vi "drop_chunks.vi"(5 "hyper_table_name":string, 7 "connection_reference":T3, 8 "error in (no error)":errorcluster, 9 "chunk_options":T2 {"newer_than" format="%<%H:%M:%S>t"}, 10 "older_than":dbl format="%<%H:%M:%S>t", 11 "time_type":T1=enum."interval") -> (0 "error out":errorcluster, 3 "chunks_dropped []":string[](array[string]))   [LabVIEW 2015, in "lv-timescaledb.lvlib"]
uses:
  lv-timescaledb.lvlib
  <vilib>/addons/database/Connection.llb/Conn ObjectReference.ctl
  _controls/drop_chunk_options.ctl
  _controls/time_type.ctl
  <vilib>/addons/database/Command.llb/Cmd Execute.vi
  <vilib>/addons/database/Recordset.llb/Rec Fetch Recordset Data (CR).vi
  <vilib>/addons/database/Recordset.llb/Rec Destroy - Command.vi
  <vilib>/addons/database/Command.llb/Cmd Delete.vi
  <vilib>/addons/database/NI_Database_API.lvlib
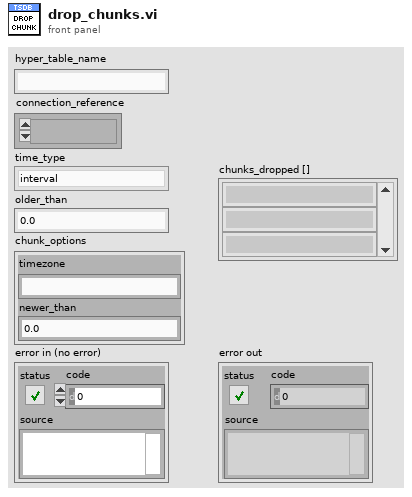
[diagram p1: front panel]
types:
  T1 = typedef "lv-timescaledb.lvlib/time_type.ctl" = enum16{"<time_type>", "interval", "timestamp", "timestamp_with_timezone", "<null>"}
  T2 = typedef "lv-timescaledb.lvlib/drop_chunk_options.ctl" = cluster{"timezone":string, "newer_than":dbl}
  T3 = typedef "NI_Database_API.lvlib/Conn ObjectReference.ctl" = refnum<k1>
  T4 = typedef "NI_Database_API.lvlib/DB Tools Parameter Info.ctl" = cluster{"parameter name":string, "type":T5, "direction":T6, "value":variant}
  T5 = typedef "NI_Database_API.lvlib/DB Tools DataTypes.ctl" = enum16{"String", "Long (I32)", "Single (SGL)", "Double (DBL)", "Date/Time", "Binary"}
  T6 = typedef "NI_Database_API.lvlib/DB Tools Parameter Dir.ctl" = enum32{"Input", "Output", "Input/Output", "Return Value"}
  T7 = cluster{"timezone":string, "postgres_date":string}
  T8 = typedef "NI_Database_API.lvlib/Cmd ObjectReference.ctl" = refnum<k1>
  T9 = typedef "NI_Database_API.lvlib/Cmd-Rec Object Reference.ctl" = refnum<k1>
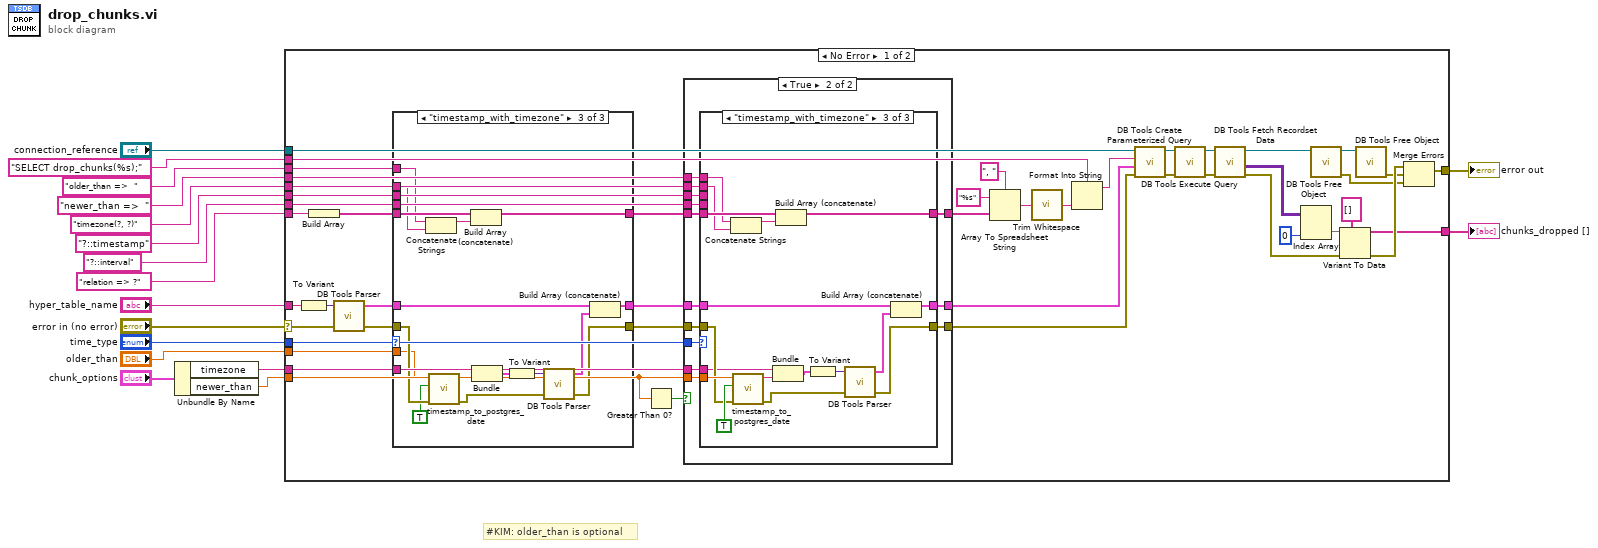
[diagram p0: block diagram]
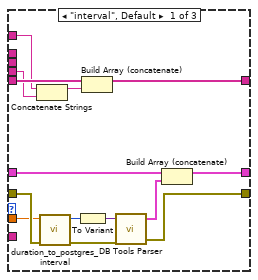
[diagram p2: hidden frame]
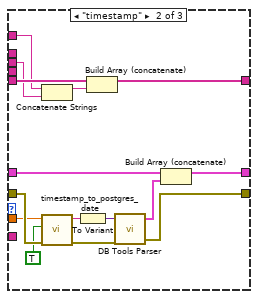
[diagram p3: hidden frame]
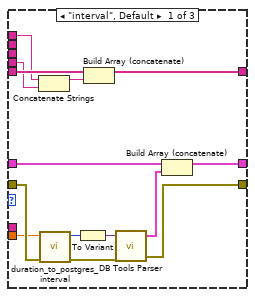
[diagram p5: hidden frame]
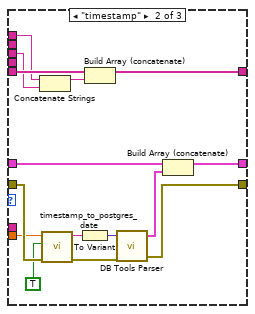
[diagram p6: hidden frame]
diagram:
  # "#KIM: older_than is optional"
  n1 = Unbundle By Name("chunk_options") -> ("timezone"=w1:string, "newer_than"=w9:dbl)
  n2 = case shown="No Error" "error in (no error)" {
    selector: "error in (no error)" -> [w45 w172]
    tunnel: "connection_reference" -> [w50 _]
    tunnel: [w61 w172] -> w15
    tunnel: [w47 _] -> w14
    tunnel: "hyper_table_name" -> [w44 _]
    tunnel: "time_type" -> [w25 _]
    tunnel: "older_than" -> [w40 _]
    tunnel: w9 -> [w32 _]
    tunnel: "SELECT drop_chunks(%s);" -> [w39 _]
    tunnel: "relation => ?" -> [w31 _]
    tunnel: "?::interval" -> [w20 _]
    tunnel: "?::timestamp" -> [w22 _]
    tunnel: "timezone(?, ?)" -> [w19 _]
    tunnel: "newer_than =>  " -> [w23 _]
    tunnel: "older_than =>  " -> [w24 _]
    tunnel: w1 -> [w18 _]
    frame No Error {
      n3 = To Variant(anything=w44) -> (Variant=w43:variant)
      n4 = Build Array(w31) -> (w30:string[])
      n5 = call <vilib>:"DB Tools Parser.vi"("error in (no error)"=w45, "variant"=w43) -> ("error out"=w41:errorcluster, "parameters"=w42:T4[])  [unwired: 2 in]
      n6 = case shown="\"timestamp_with_timezone\"" w25 {
        tunnel: w42 -> [w72 w84 w102]
        tunnel: w41 -> [w77 w92 w109]
        tunnel: w40 -> [w76 w91 w108]
        tunnel: [w71 w85 w103] -> w34
        tunnel: [w69 w83 w101] -> w63
        tunnel: w30 -> [w68 w81 w99]
        tunnel: [w67 w80 w98] -> w29
        tunnel: w24 -> [w64 w79 w97]
        tunnel: w20 -> [w65 _ _]
        tunnel: w22 -> [_ w78 _]
        tunnel: w18 -> [_ _ w93]
        tunnel: w19 -> [_ _ w96]
        frame "interval", Default {
          n7 = Concatenate Strings(w64, w65) -> (w66:string)
          n8 = call "duration_to_postgres_interval.vi"("error in (no error)"=w77, "interval"=w76) -> ("error out"=w74:errorcluster, "millisecond"=w75:i32)  [unwired: 8 in]
          n9 = To Variant(anything=w75) -> (Variant=w73:variant)
          n10 = Build Array (concatenate)(w68, w66) -> (w67:string[])
          n11 = call <vilib>:"DB Tools Parser.vi"("error in (no error)"=w74, "variant"=w73) -> ("error out"=w69:errorcluster, "parameters"=w70:T4[])  [unwired: 2 in]
          n12 = Build Array (concatenate)(w72, w70) -> (w71:T4[])
        }
        frame "timestamp" {
          n13 = Concatenate Strings(w79, w78) -> (w82:string)
          n14 = call "timestamp_to_postgres_date.vi"("error in (no error)"=w92, "utc"=TRUE, "date_time"=w91) -> ("error out"=w88:errorcluster, "postgres_date"=w89:string)  [unwired: 7 in]
          n15 = To Variant(anything=w89) -> (Variant=w87:variant)
          n16 = Build Array (concatenate)(w81, w82) -> (w80:string[])
          n17 = call <vilib>:"DB Tools Parser.vi"("error in (no error)"=w88, "variant"=w87) -> ("error out"=w83:errorcluster, "parameters"=w86:T4[])  [unwired: 2 in]
          n18 = Build Array (concatenate)(w84, w86) -> (w85:T4[])
        }
        frame "timestamp_with_timezone" {
          n19 = Concatenate Strings(w97, w96) -> (w100:string)
          n20 = call "timestamp_to_postgres_date.vi"("error in (no error)"=w109, "utc"=TRUE, "date_time"=w108) -> ("error out"=w106:errorcluster, "postgres_date"=w94:string)  [unwired: 7 in]
          n21 = Build Array (concatenate)(w99, w100) -> (w98:string[])
          n22 = Bundle("timezone"=w93, "postgres_date"=w94) -> (w95:T7)  [unwired: 1 in]
          n23 = To Variant(anything=w95) -> (Variant=w105:variant)
          n24 = call <vilib>:"DB Tools Parser.vi"("error in (no error)"=w106, "variant"=w105) -> ("error out"=w101:errorcluster, "parameters"=w104:T4[])  [unwired: 2 in]
          n25 = Build Array (concatenate)(w102, w104) -> (w103:T4[])
        }
      }
      n26 = Greater Than 0?(x=w32) -> (x > 0?=w27:bool)
      n27 = case shown="True" w27 {
        tunnel: w25 -> [_ w125]
        tunnel: w34 -> [w111 w124]
        tunnel: [w111 w123] -> w33
        tunnel: w63 -> [w110 w122]
        tunnel: w32 -> [_ w121]
        tunnel: w29 -> [w112 w120]
        tunnel: [w112 w116] -> w28
        tunnel: [w110 w119] -> w26
        tunnel: w23 -> [_ w118]
        tunnel: w22 -> [_ w117]
        tunnel: w20 -> [_ w115]
        tunnel: w19 -> [_ w114]
        tunnel: w18 -> [_ w113]
        frame False {
        }
        frame True {
          n28 = case shown="\"timestamp_with_timezone\"" w125 {
            tunnel: w121 -> [w138 w153 w171]
            tunnel: [w134 w147 w166] -> w123
            tunnel: [w127 w146 w165] -> w119
            tunnel: w124 -> [w128 w145 w163]
            tunnel: w122 -> [w139 w154 w164]
            tunnel: w120 -> [w131 w143 w161]
            tunnel: w118 -> [w129 w142 w160]
            tunnel: w117 -> [_ w140 _]
            tunnel: [w130 w141 w159] -> w116
            tunnel: w115 -> [w126 _ _]
            tunnel: w114 -> [_ _ w158]
            tunnel: w113 -> [_ _ w155]
            frame "interval", Default {
              n29 = Concatenate Strings(w129, w126) -> (w132:string)
              n30 = call "duration_to_postgres_interval.vi"("error in (no error)"=w139, "interval"=w138) -> ("error out"=w136:errorcluster, "millisecond"=w137:i32)  [unwired: 8 in]
              n31 = To Variant(anything=w137) -> (Variant=w135:variant)
              n32 = Build Array (concatenate)(w131, w132) -> (w130:string[])
              n33 = call <vilib>:"DB Tools Parser.vi"("error in (no error)"=w136, "variant"=w135) -> ("error out"=w127:errorcluster, "parameters"=w133:T4[])  [unwired: 2 in]
              n34 = Build Array (concatenate)(w128, w133) -> (w134:T4[])
            }
            frame "timestamp" {
              n35 = Concatenate Strings(w142, w140) -> (w144:string)
              n36 = call "timestamp_to_postgres_date.vi"("error in (no error)"=w154, "utc"=TRUE, "date_time"=w153) -> ("error out"=w150:errorcluster, "postgres_date"=w151:string)  [unwired: 7 in]
              n37 = To Variant(anything=w151) -> (Variant=w149:variant)
              n38 = Build Array (concatenate)(w143, w144) -> (w141:string[])
              n39 = call <vilib>:"DB Tools Parser.vi"("error in (no error)"=w150, "variant"=w149) -> ("error out"=w146:errorcluster, "parameters"=w148:T4[])  [unwired: 2 in]
              n40 = Build Array (concatenate)(w145, w148) -> (w147:T4[])
            }
            frame "timestamp_with_timezone" {
              n41 = Concatenate Strings(w160, w158) -> (w162:string)
              n42 = call "timestamp_to_postgres_date.vi"("error in (no error)"=w164, "utc"=TRUE, "date_time"=w171) -> ("error out"=w169:errorcluster, "postgres_date"=w157:string)  [unwired: 7 in]
              n43 = Bundle("timezone"=w155, "postgres_date"=w157) -> (w156:T7)  [unwired: 1 in]
              n44 = Build Array (concatenate)(w161, w162) -> (w159:string[])
              n45 = To Variant(anything=w156) -> (Variant=w168:variant)
              n46 = call <vilib>:"DB Tools Parser.vi"("error in (no error)"=w169, "variant"=w168) -> ("error out"=w165:errorcluster, "parameters"=w167:T4[])  [unwired: 2 in]
              n47 = Build Array (concatenate)(w163, w167) -> (w166:T4[])
            }
          }
        }
      }
      n48 = Array To Spreadsheet String(delimiter (Tab)=", ", array=w28, 3:"%s" ("format string")) -> (spreadsheet string=w36:string)
      n49 = call <vilib>:"Trim Whitespace.vi"("string"=w36) -> ("trimmed string"=w21:string)  [unwired: 1 in]
      n50 = Format Into String(format string=w39, w21) -> (resulting string=w38:string)  [unwired: 2 in, 1 out]
      n51 = call <vilib>:"DB Tools Create Parameterized Query.vi"("error in (no error)"=w26, "parameters"=w33, "SQL query"=w38, "connection reference"=w50) -> ("error out"=w55:errorcluster, "command reference"=w56:T8)  [unwired: 3 in, 1 out]
      n52 = call-poly <vilib>:"DB Tools Execute Query.vi"("error in (no error)"=w55, "command reference"=w56) -> ("error out"=w52:errorcluster, "command-recordset reference"=w54:T9)  [unwired: 6 in]
      n53 = call-poly <vilib>:"DB Tools Fetch Recordset Data.vi"("error in (no error)"=w52, "command-recordset reference"=w54) -> ("error out"=w58:errorcluster, "recordset data"=w59:variant[][], "command-recordset reference out"=w53:T9)  [unwired: 3 in]
      n54 = Index Array(array=w59, index (col)=0 ("disabled index (col)")) -> (element=w46:variant[])  [unwired: 1 in]
      n55 = call-poly <vilib>:"DB Tools Free Object.vi"("command-recordset reference"=w53) -> ("error out"=w49:errorcluster, "command reference"=w57:T8)  [unwired: 9 in]
      n56 = Variant To Data(error in=w58, type=string[] [] ("Array"), Variant=w46) -> (data=w47:string[], error out=w62:errorcluster)
      n57 = call-poly <vilib>:"DB Tools Free Object.vi"("command reference"=w57) -> ("error out"=w51:errorcluster)  [unwired: 9 in, 1 out]
      n58 = Merge Errors(w62, w51, w49) -> (w61:errorcluster)
    }
    frame Error {
    }
  }
  "error out" <- w15
  "chunks_dropped []" <- w14
